vi "showPosition.vi"(8 "error in (no error)":errorcluster, 11 "Cell in":refnum<class "Cell.lvclass">) -> (0 "error out":errorcluster)   [LabVIEW 2014, in "Cell.lvclass"]
uses:
  Cell.lvclass
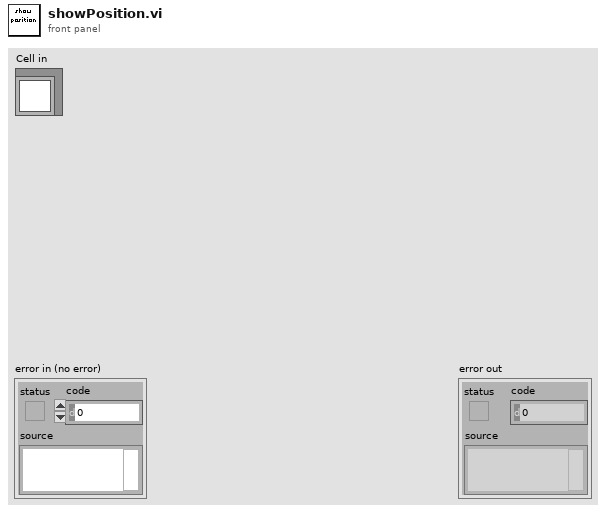
[diagram p1: front panel]
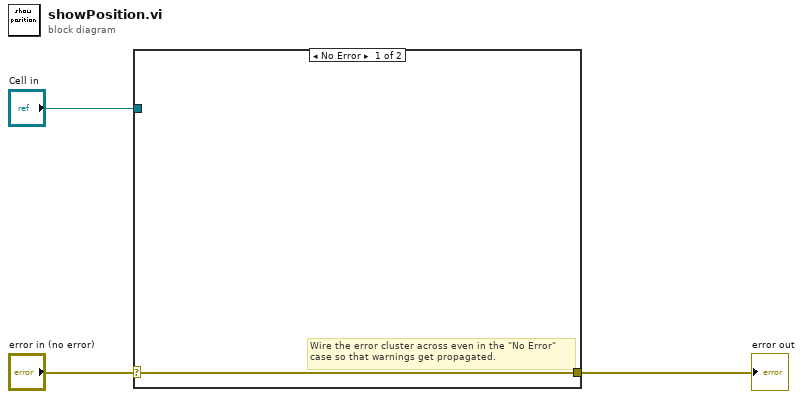
[diagram p0: block diagram]
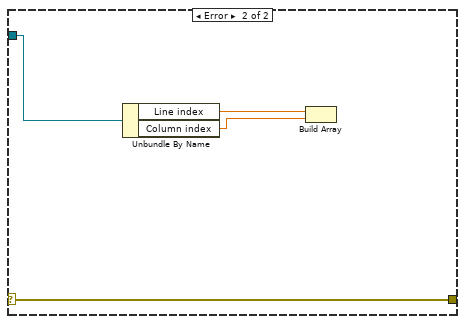
[diagram p2: hidden frame]
diagram:
  n1 = case shown="No Error" "error in (no error)" {
    selector: "error in (no error)" -> [w4 w9]
    tunnel: [w4 w9] -> w2
    tunnel: "Cell in" -> [_ w8]
    frame No Error {
      # "Wire the error cluster across even in the \"No Error\"\ncase so that warnings get propagated."
    }
    frame Error {
      n2 = Unbundle By Name(w8) -> ("Line index"=w7:dbl, "Column index"=w6:dbl)
      n3 = Build Array(w7, w6) -> (w5:dbl[])
    }
  }
  "error out" <- w2
